vi "util_set_change_out.vi"(7 "references":T1, 8 "error in (no error)":errorcluster, 10 "data":variant, 11 "change":bool) -> (0 "error out":errorcluster)   [LabVIEW 2015, in "repub-dvr_nre.lvlib"]
uses:
  repub-dvr_nre.lvlib
  public/_controls/references.ctl
  _controls/input.ctl
  _controls/input_command.ctl
  _controls/output.ctl
  _controls/data.ctl
  public/_controls/configuration.ctl
  lv-recipe-machine/private/_controls/recipe_data.ctl
  lv-recipe-machine/public/_controls/mode.ctl
  lv-recipe-machine/public/_controls/manual_state.ctl
  lv-recipe-machine/public/_controls/automatic_state.ctl
  <userlib>/antonio-alexander/lv-waitgroup/public/_controls/api_waitgroup.ctl
  lv-recipe-machine/public/_controls/transition.ctl
  public/_controls/change.ctl
  public/_controls/status.ctl
  lv-recipe-machine/lv-recipe-machine.lvlib
  <userlib>/antonio-alexander/lv-waitgroup/lv-waitgroup.lvlib
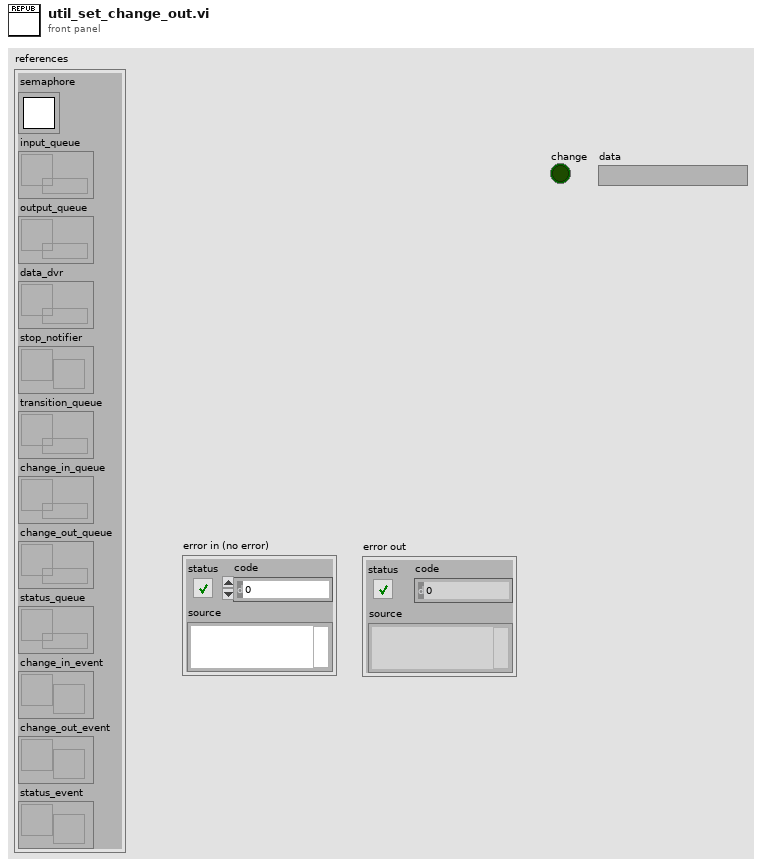
[diagram p1: front panel]
types:
  T1 = typedef "repub-dvr_nre.lvlib/references.ctl" = cluster{"semaphore":T2, "input_queue":refnum<queue>, "output_queue":refnum<queue>, "data_dvr":refnum<data-value>, "stop_notifier":refnum<notifier>, "transition_queue":refnum<queue>, "change_in_queue":refnum<queue>, "change_out_queue":refnum<queue>, "status_queue":refnum<queue>, "change_in_event":refnum<user-event>, "change_out_event":refnum<user-event>, "status_event":refnum<user-event>}
  T2 = typedef "Semaphore RefNum" = refnum<k1>
  T3 = typedef "repub-dvr_nre.lvlib/change.ctl" = cluster{"changed":bool, "data":variant}
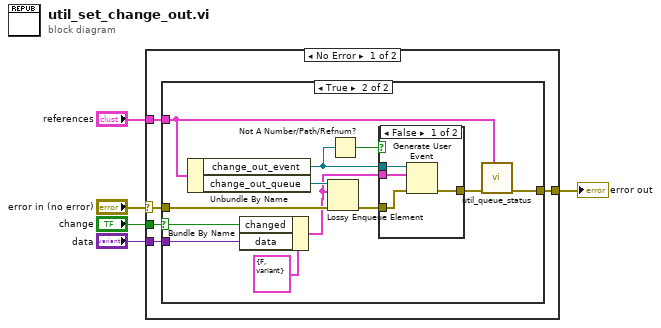
[diagram p0: block diagram]
diagram:
  n1 = case shown="No Error" "error in (no error)" {
    selector: "error in (no error)" -> [w9 w29]
    tunnel: [w6 w29] -> w4
    tunnel: "references" -> [w10 _]
    tunnel: "change" -> [w8 _]
    tunnel: "data" -> [w7 _]
    frame No Error {
      n2 = case shown="True" w8 {
        selector: w8 -> [_ w20]
        tunnel: w10 -> [_ w14]
        tunnel: w9 -> [w11 w22]
        tunnel: w7 -> [_ w19]
        tunnel: [w11 w12] -> w6
        frame False {
        }
        frame True {
          n3 = Unbundle By Name(w14) -> ("change_out_event"=w17:refnum<user-event>, "change_out_queue"=w23:refnum<queue>)
          n4 = Bundle By Name(cluster=T3 {"changed"=FALSE, "data"=variant} ("change"), "changed"=w20, "data"=w19) -> (w15:T3)
          n5 = Lossy Enqueue Element(queue=w23, element=w15, error in (no error)=w22) -> (error out=w16:errorcluster)  [unwired: 3 out]
          n6 = Not A Number/Path/Refnum?(number/path/refnum=w17) -> (NaN/Path/Refnum?=w18:bool)
          n7 = case shown="False" w18 {
            tunnel: w15 -> [w27 _]
            tunnel: w16 -> [w26 w28]
            tunnel: [w25 w28] -> w13
            tunnel: w17 -> [w24 _]
            frame False {
              n8 = Generate User Event(user event=w24, event data cluster=w27, error in=w26) -> (error out=w25:errorcluster)  [unwired: 1 in, 1 out]
            }
            frame True {
            }
          }
          n9 = call "util_queue_status.vi"("references"=w14, "error in (no error)"=w13) -> ("error out"=w12:errorcluster)  [unwired: 9 in]
        }
      }
    }
    frame Error {
    }
  }
  "error out" <- w4
